vi "ACal-Update In Ear Parameters.vi"(0 "Params in":T1 {"Weighted"."WF" items=["Chirp", "Noise"]}, 5 "Section":string) -> (4 "Params out":T1 {"Weighted"."WF" items=["Chirp", "Noise"]})   [LabVIEW 2020]
uses:
  Type Defs/ACal-In Ear Parameters.ctl
  epl-vi-lib/Utility VIs/Type Defs/Speaker ring.ctl
  Type Defs/Cal Stimulus.ctl
  Type Defs/ACal-Multiband Parameters.ctl
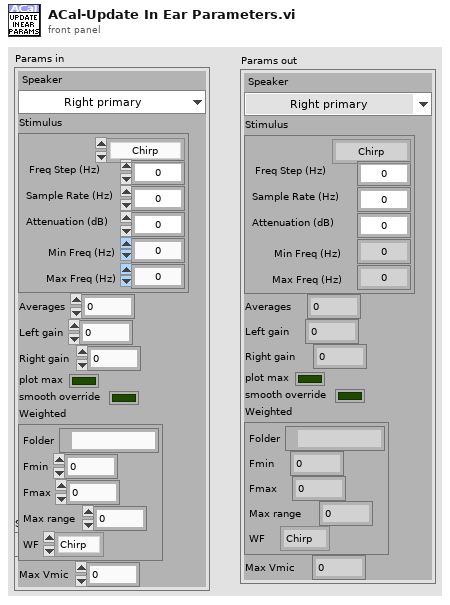
[diagram p1: front panel]
types:
  T1 = typedef "ACal-In Ear Parameters.ctl" = cluster{"Speaker":T2, "Stimulus":T3, "Averages":i32, "Left gain":dbl, "Right gain":dbl, "plot max":bool, "smooth override":bool, "Weighted":T4, "Max Vmic":dbl}
  T2 = typedef "Speaker ring.ctl" = enum16{"Right primary", "Right secondary", "Left primary", "Left secondary"}
  T3 = typedef "Cal Stimulus.ctl" = cluster{"Min Freq (Hz)":dbl, "Max Freq (Hz)":dbl, "Freq Step (Hz)":dbl, "Waveform":enum16{"Chirp", "Weighted"}, "Attenuation (dB)":dbl, "Sample Rate (Hz)":dbl}
  T4 = typedef "ACal-Multiband Parameters.ctl" = cluster{"Folder":path, "Fmin":dbl, "Fmax":dbl, "Max range":dbl, "WF":u16}
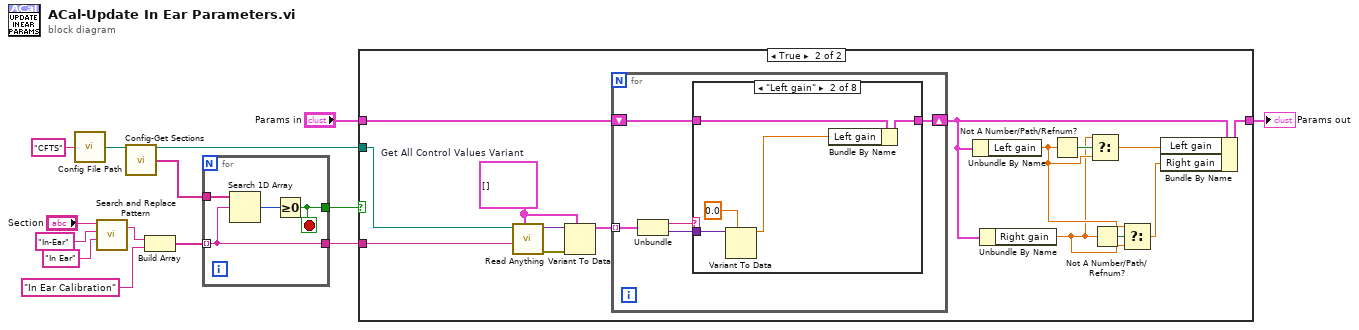
[diagram p0: block diagram]
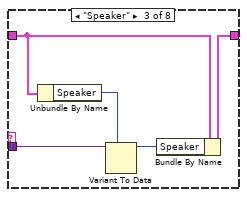
[diagram p4: hidden frame]
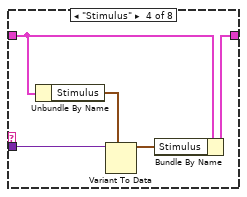
[diagram p5: hidden frame]
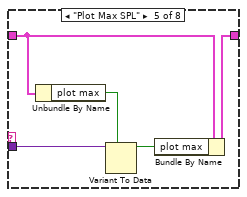
[diagram p6: hidden frame]
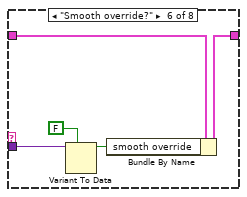
[diagram p7: hidden frame]
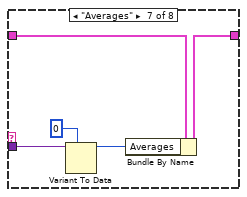
[diagram p8: hidden frame]
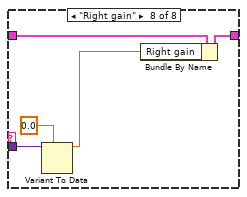
[diagram p9: hidden frame]
diagram:
  n1 = call "Config File Path.vi"("AppName"="CFTS") -> ("Default config file name"=w12:path)
  n2 = call <vilib>:"Search and Replace Pattern.vi"("string"="Section", "regular expression (\"\")"="In-Ear" ("regular expression (\"\")"), "replace string (\"\")"="In Ear" ("replace string (\"\")")) -> ("result string"=w4:string)  [unwired: 2 in, 1 out]
  n3 = call "Config-Get Sections.vi"("configuration file path"=w12) -> ("file path"=w7:path, "section names"=w10:string[])  [unwired: 12 in, 1 out]
  n4 = Build Array(w4, "In Ear Calibration" ("element")) -> (w11:string[])
  n5 = for {
    tunnel: w11 -> [w15] mode=indexing
    tunnel: w10 -> [w18]
    tunnel: [w16] -> w9
    tunnel: [w15] -> w8
    stop <- w16 stop-if-true
    n6 = Search 1D Array(1D array=w18, element=w15) -> (index of element=w17:i32)  [unwired: 1 in]
    n7 = Greater Or Equal To 0?(x=w17) -> (x >= 0?=w16:bool)
  }
  n8 = case shown="True" w9 {
    tunnel: w8 -> [_ w34]
    tunnel: w7 -> [_ w33]
    tunnel: "Params in" -> [w19 w32]
    tunnel: [w19 w26] -> w5
    frame False {
    }
    frame True {
      w29 = cluster{"Name":string, "Variant Data":variant}[] []  # Get All Control Values Variant
      n9 = call "Read Anything.vi"("Type of Anything"=w29, "Section Name (Name of \"Type of Anything\")"=w34, "Path (dialog)"=w33) -> ("Error Out"=w31:errorcluster, "Anything"=w30:variant)  [unwired: 1 in, 6 out]
      n10 = Variant To Data(error in=w31, type=w29, Variant=w30) -> (data=w28:cluster{"Name":string, "Variant Data":variant}[])  [unwired: 1 out]
      n11 = for {
        shift-right: [w38] -> w27
        shift-left: w32 -> [w37]
        tunnel: w28 -> [w39] mode=indexing
        n12 = Unbundle(w39) -> ("Name"=w36:string, "Variant Data"=w35:variant)
        n13 = case shown="\"Left gain\"" w36 {
          tunnel: [w40 w42 w49 w54 w59 w64 w69 w72] -> w38
          tunnel: w37 -> [w40 w45 w47 w52 w57 w62 w67 w75]
          tunnel: w35 -> [_ w44 w50 w55 w60 w65 w70 w74]
          frame "", Default {
          }
          frame "Left gain" {
            n14 = Variant To Data(type=0.0, Variant=w44) -> (data=w41:dbl)  [unwired: 1 in, 1 out]
            n15 = Bundle By Name(cluster=w45, "Left gain"=w41) -> (w42:T1)
          }
          frame "Speaker" {
            n16 = Unbundle By Name(w47) -> ("Speaker"=w46:T2)
            n17 = Variant To Data(type=w46, Variant=w50) -> (data=w48:T2)  [unwired: 1 in, 1 out]
            n18 = Bundle By Name(cluster=w47, "Speaker"=w48) -> (w49:T1)
          }
          frame "Stimulus" {
            n19 = Unbundle By Name(w52) -> ("Stimulus"=w51:T3)
            n20 = Variant To Data(type=w51, Variant=w55) -> (data=w53:T3)  [unwired: 1 in, 1 out]
            n21 = Bundle By Name(cluster=w52, "Stimulus"=w53) -> (w54:T1)
          }
          frame "Plot Max SPL" {
            n22 = Unbundle By Name(w57) -> ("plot max"=w56:bool)
            n23 = Variant To Data(type=w56, Variant=w60) -> (data=w58:bool)  [unwired: 1 in, 1 out]
            n24 = Bundle By Name(cluster=w57, "plot max"=w58) -> (w59:T1)
          }
          frame "Smooth override?" {
            n25 = Variant To Data(type=FALSE, Variant=w65) -> (data=w63:bool)  [unwired: 1 in, 1 out]
            n26 = Bundle By Name(cluster=w62, "smooth override"=w63) -> (w64:T1)
          }
          frame "Averages" {
            n27 = Variant To Data(type=0, Variant=w70) -> (data=w68:i32)  [unwired: 1 in, 1 out]
            n28 = Bundle By Name(cluster=w67, "Averages"=w68) -> (w69:T1)
          }
          frame "Right gain" {
            n29 = Variant To Data(type=0.0, Variant=w74) -> (data=w71:dbl)  [unwired: 1 in, 1 out]
            n30 = Bundle By Name(cluster=w75, "Right gain"=w71) -> (w72:T1)
          }
        }
      }
      n31 = Unbundle By Name(w27) -> ("Left gain"=w22:dbl)
      n32 = Unbundle By Name(w27) -> ("Right gain"=w21:dbl)
      n33 = Not A Number/Path/Refnum?(number/path/refnum=w22) -> (NaN/Path/Refnum?=w25:bool)
      n34 = Select(t=w21, s=w25, f=w22) -> (s? t:f=w24:dbl)
      n35 = Not A Number/Path/Refnum?(number/path/refnum=w21) -> (NaN/Path/Refnum?=w23:bool)
      n36 = Select(t=w22, s=w23, f=w21) -> (s? t:f=w20:dbl)
      n37 = Bundle By Name(cluster=w27, "Left gain"=w24, "Right gain"=w20) -> (w26:T1)
    }
  }
  "Params out" <- w5
